vi "ReproducirSenalDTMF.vi"(2 "Min_Frecuencia":dbl, 3 "Max_Frecuencia":dbl) -> ()   [LabVIEW 2018]
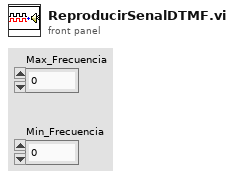
[diagram p1: front panel]
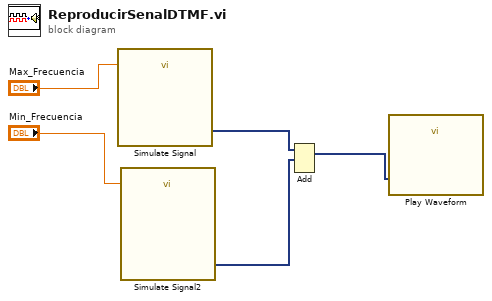
[diagram p0: block diagram]
diagram:
  n1 = call "Simulate Signal"("Frequency"="Max_Frecuencia") -> ("Sine"=w3:dynamicdata)  [unwired: 13 in, 1 out]
  n2 = call "Simulate Signal2"("Frequency"="Min_Frecuencia") -> ("Sine"=w2:dynamicdata)  [unwired: 13 in, 1 out]
  n3 = Add(1:w2, 2:w3) -> (0:w1:dynamicdata)  [unwired: 1 in, 1 out]
  n4 = call "Play Waveform"("Data"=w1) -> ()  [unwired: 18 in, 1 out]
